vi "RemoveProject.vi"(8 "error in (no error)":errorcluster, 11 "Project.lvclass In":refnum<class "Project.lvclass">) -> (0 "error out":errorcluster, 2 "ProjectSelectIdx":i32, 3 "Project.lvclass Out":refnum<class "Project.lvclass">)   [LabVIEW 2014, in "Project.lvclass"]
uses:
  Project.lvclass
  Project.lvclass/Project.ctl
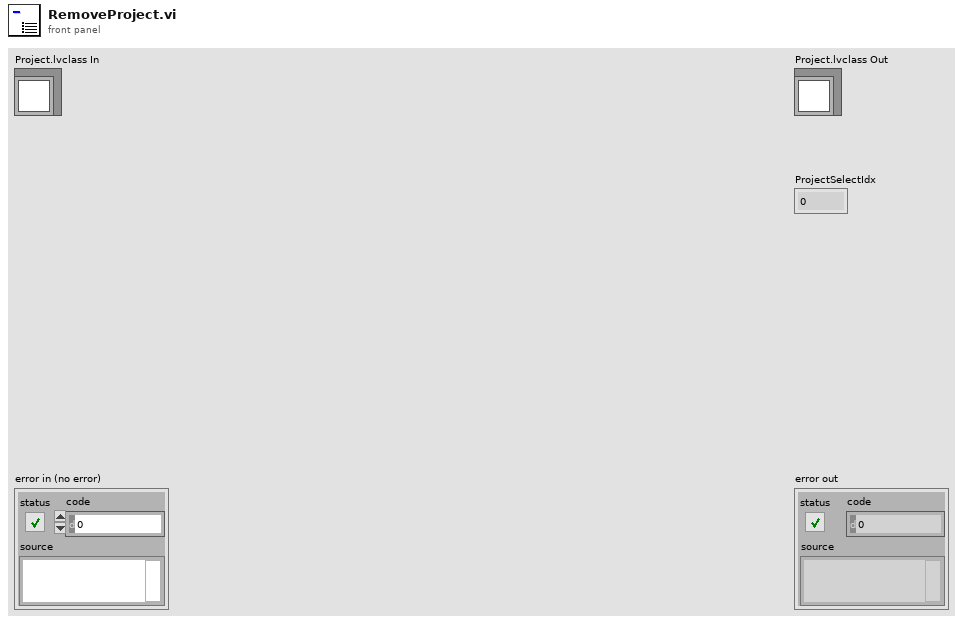
[diagram p1: front panel]
types:
  T1 = typedef "Project.lvclass/ProjectDataTableTypeDefine.ctl" = string[][]
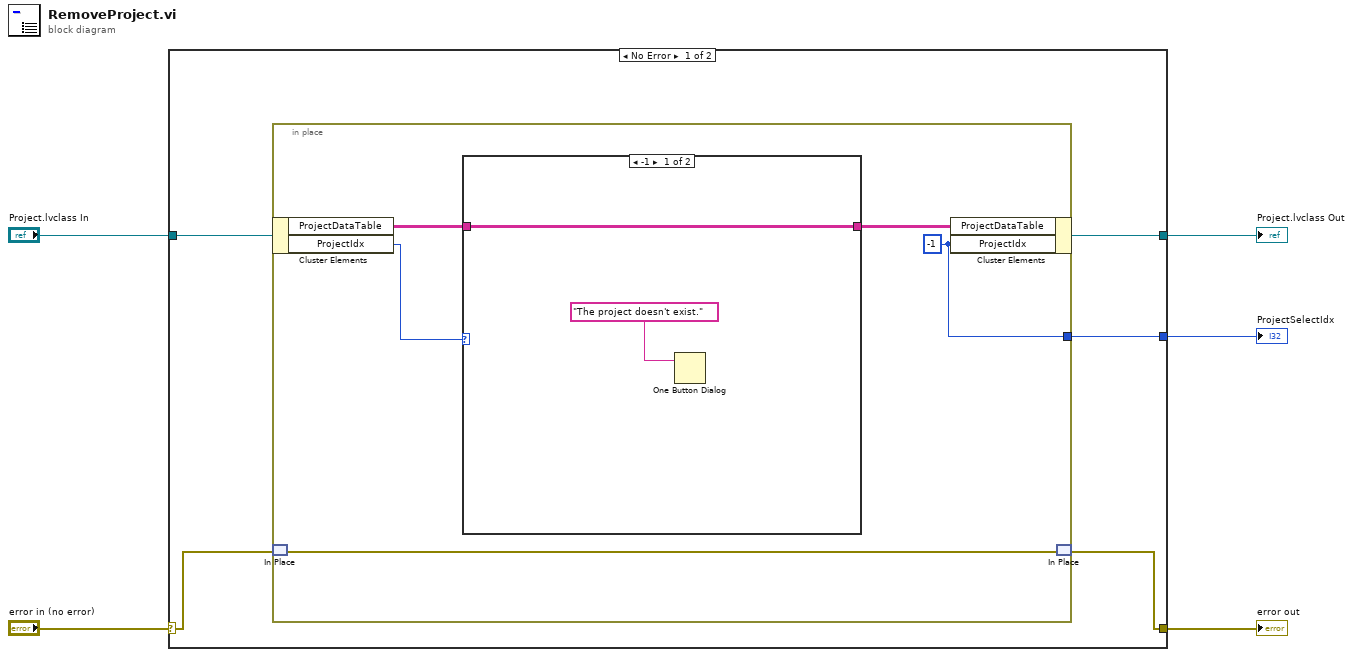
[diagram p0: block diagram]
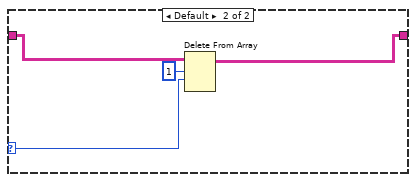
[diagram p2: hidden frame]
diagram:
  n1 = case shown="No Error" "error in (no error)" {
    selector: "error in (no error)" -> [w10 w23]
    tunnel: [w6 w23] -> w4
    tunnel: "Project.lvclass In" -> [w9 w22]
    tunnel: [w8 w22] -> w2
    tunnel: [w7 _] -> w1
    frame No Error {
      n2 = in-place {
        in-place-border: [w12] -> w7
        w12 = -1 ("ProjectIdx")
        n3 = in-place-cluster #1(w9) -> ("ProjectDataTable"=w15:T1, "ProjectIdx"=w14:i32)
        n4 = in-place-match #2(w10) -> (w11:errorcluster)
        n5 = case shown="-1" w14 {
          selector: w14 -> [_ w18]
          tunnel: w15 -> [w17 w21]
          tunnel: [w17 w20] -> w13
          frame -1 {
            n6 = One Button Dialog(message="The project doesn't exist.") -> ()  [unwired: 1 in, 1 out]
          }
          frame Default {
            n7 = Delete From Array(array=w21, length=1, index (row)=w18) -> (array with subset deleted=w20:T1)  [unwired: 1 in, 1 out]
          }
        }
        n8 = in-place-cluster #1("ProjectDataTable"=w13, "ProjectIdx"=w12) -> (w8:refnum<class "Project.lvclass">)
        n9 = in-place-match #2(w11) -> (w6:errorcluster)
      }
    }
    frame Error {
    }
  }
  "error out" <- w4
  "Project.lvclass Out" <- w2
  "ProjectSelectIdx" <- w1
